vi "stop.vi"(3 "error in (no error)":errorcluster, 4 "stop":bool, 5 "HamegHMPSupply in":refnum<class "HamegHMPSupply.lvclass">) -> (0 "error out":errorcluster, 1 "Stopped":bool, 2 "HamegHMPSupply out":refnum<class "HamegHMPSupply.lvclass">)   [LabVIEW 2011, in "Hardware.lvlib" / "Channels.lvlib" / "HamegHMPSupply.lvclass"]
doc: "Abstract Method.\n\nStops the analog output. This vi indicates of the analog output has stopped, and can be used to actively stop the output."
uses:
  HamegHMPSupply.lvclass
  HamegHMPSupply.lvclass/HamegHMPSupply.ctl
  AnalogOutput.lvclass
  Tools/Filing/FileNeologist/FileNeologist.lvclass
  Tools/Filing.lvlib
panel:
  in  "measure":bool=TRUE
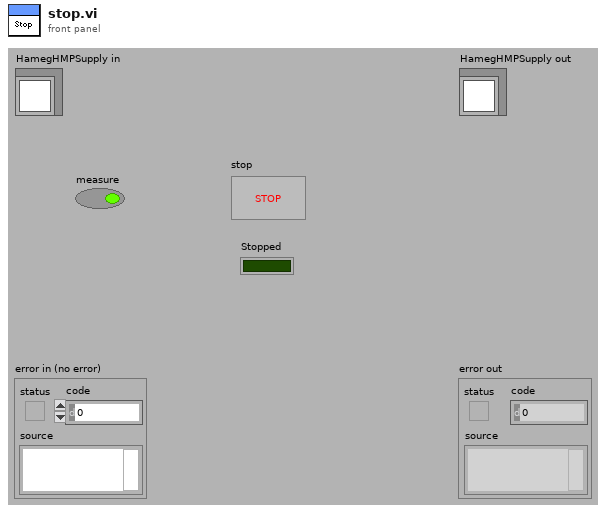
[diagram p1: front panel]
types:
  T1 = enum16{"open", "replace", "create", "open or create", "replace or create", "replace or create with confirmation"}
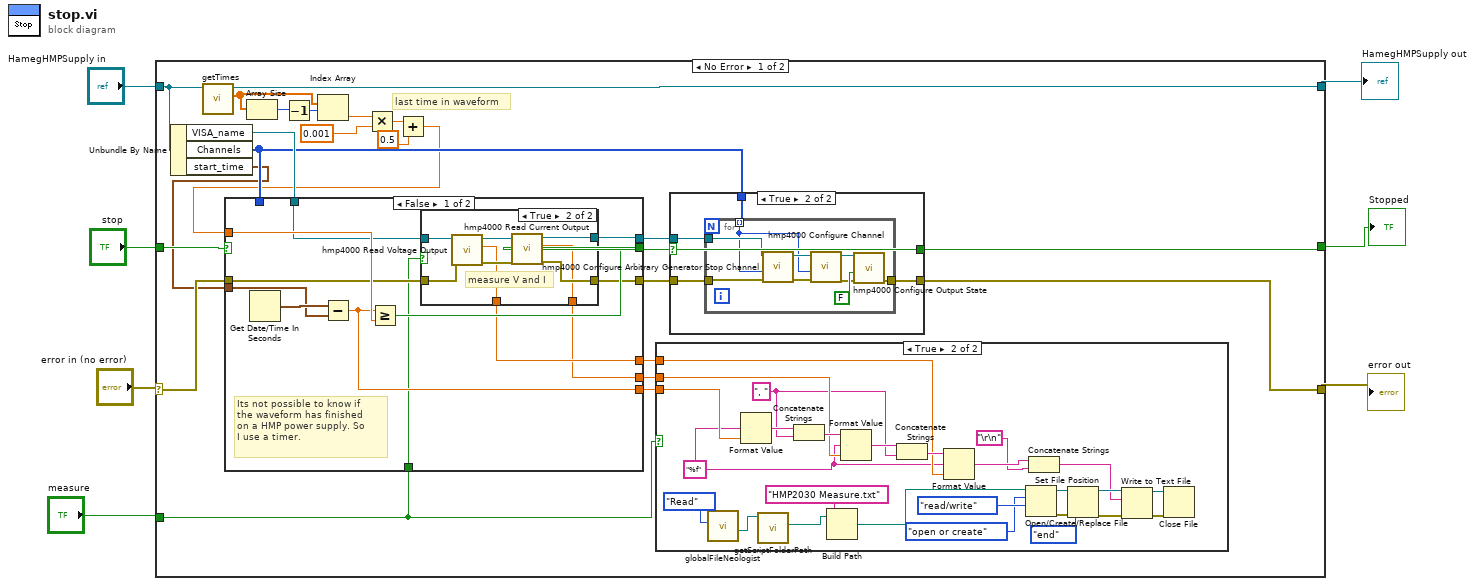
[diagram p0: block diagram]
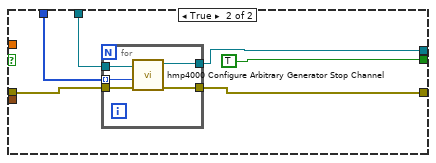
[diagram p5: hidden frame]
diagram:
  n1 = case shown="No Error" "error in (no error)" {
    selector: "error in (no error)" -> [w29 w107]
    tunnel: [w21 w109] -> w7
    tunnel: "HamegHMPSupply in" -> [w22 w109]
    tunnel: [w25 w107] -> w2
    tunnel: [w24 w108] -> w4
    tunnel: "stop" -> [w30 w108]
    tunnel: "measure" -> [w8 _]
    frame No Error {
      # "last time in waveform"
      n2 = Unbundle By Name(w22) -> ("VISA_name"=w31:refnum<visa-resource-name>, "Channels"=w23:i32[], "start_time"=w12:timestamp)
      n3 = call "getTimes.vi"("AnalogOutput in"=w22) -> ("times"=w18:dbl[], "AnalogOutput out"=w21:refnum<class "HamegHMPSupply.lvclass">)  [unwired: 8 in, 1 out]
      n4 = Array Size(array=w18) -> (size(s)=w20:i32)
      n5 = Decrement(x=w20) -> (x-1=w19:i32)
      n6 = Index Array(array=w18, index=w19) -> (element=w17:dbl)
      n7 = Multiply(x=w17, y=0.001) -> (x*y=w16:dbl)
      n8 = Add(x=w16, y=0.5) -> (x+y=w13:dbl)
      n9 = case shown="False" w30 {
        tunnel: w31 -> [w81 w101]
        tunnel: [w82 TRUE] -> w28
        tunnel: w23 -> [_ w100]
        tunnel: [w79 w99] -> w27
        tunnel: w29 -> [w78 w98]
        tunnel: [w80 w96] -> w26
        tunnel: w13 -> [w83 _]
        tunnel: w12 -> [w84 _]
        tunnel: [w77 _] -> w9
        tunnel: [w76 _] -> w10
        tunnel: [w75 _] -> w11
        tunnel: w8 -> [w74 _]
        frame False {
          # "Its not possible to know if\nthe waveform has finished\non a HMP power supply. So \nI use a timer."
          n10 = Get Date/Time In Seconds() -> (seconds since 1Jan1904=w85:timestamp)
          n11 = Subtract(x=w85, y=w84) -> (x-y=w75:dbl)
          n12 = Greater Or Equal?(x=w75, y=w83) -> (x >= y?=w82:bool)
          n13 = case shown="True" w74 {
            tunnel: w81 -> [w86 w93]
            tunnel: [w86 w92] -> w80
            tunnel: [w87 w91] -> w79
            tunnel: w78 -> [w87 w90]
            tunnel: [_ w89] -> w77
            tunnel: [_ w88] -> w76
            frame False {
            }
            frame True {
              # "measure V and I"
              n14 = call <instrlib>:"hmp4000 Read Voltage Output.vi"("error in (no error)"=w90, "VISA resource name"=w93) -> ("error out"=w94:errorcluster, "Voltage Value"=w89:dbl, "VISA resource name out"=w95:refnum<visa-resource-name>)  [unwired: 7 in]
              n15 = call <instrlib>:"hmp4000 Read Current Output.vi"("error in (no error)"=w94, "VISA resource name"=w95) -> ("error out"=w91:errorcluster, "Current Value"=w88:dbl, "VISA resource name out"=w92:refnum<visa-resource-name>)  [unwired: 7 in]
            }
          }
        }
        frame True {
          n16 = for {
            tunnel: w101 -> [w106]
            tunnel: w100 -> [w105] mode=indexing
            tunnel: [w104] -> w99
            tunnel: w98 -> [w103]
            tunnel: [w102] -> w96
            n17 = call <instrlib>:"hmp4000 Configure Arbitrary Generator Stop Channel.vi"("error in (no error)"=w103, "Channel (Channel 1)"=w105, "VISA resource name"=w106) -> ("error out"=w104:errorcluster, "VISA resource name out"=w102:refnum<visa-resource-name>)  [unwired: 7 in]
          }
        }
      }
      n18 = case shown="True" w8 {
        tunnel: w11 -> [_ w57]
        tunnel: w10 -> [_ w54]
        tunnel: w9 -> [_ w50]
        frame False {
        }
        frame True {
          w51 = ", "
          w49 = "%f"
          n19 = call "globalFileNeologist.vi"("Action"=enum16{"Write", "Read"}."Read") -> ("FileNeologist out"=w47:refnum<class "FileNeologist.lvclass">)  [unwired: 10 in]
          n20 = Format Value(format string=w49, value (0)=w57) -> (output string=w56:string)  [unwired: 1 in]
          n21 = call "getScriptFolderPath.vi"("FileNeologist in"=w47) -> ("Path"=w46:path)  [unwired: 8 in, 2 out]
          n22 = Concatenate Strings(w56, w51) -> (w55:string)
          n23 = Build Path(base path=w46, name or relative path="HMP2030 Measure.txt") -> (appended path=w44:path)
          n24 = Format Value(string ("")=w55, format string=w49, value (0)=w54) -> (output string=w52:string)
          n25 = Concatenate Strings(w52, w51) -> (w53:string)
          n26 = Format Value(string ("")=w53, format string=w49, value (0)=w50) -> (output string=w34:string)
          n27 = Open/Create/Replace File(file path (use dialog)=w44, operation (0:open)=T1."open or create", access (0:read/write)=enum16{"read/write", "read-only", "write-only"}."read/write") -> (refnum out=w41:refnum<file>, error out=w40:errorcluster)  [unwired: 3 in, 1 out]
          n28 = Concatenate Strings(w34, "\r\n") -> (w32:string)
          n29 = Set File Position(refnum=w41, from (0:start)=enum16{"start", "end", "current"}."end", error in=w40) -> (refnum out=w38:refnum<file>, error out=w37:errorcluster)  [unwired: 1 in]
          n30 = Write to Text File(file (use dialog)=w38, text=w32, error in=w37) -> (refnum out=w35:refnum<file>, error out=w36:errorcluster)  [unwired: 1 in, 1 out]
          n31 = Close File(refnum=w35, error in=w36) -> ()  [unwired: 2 out]
        }
      }
      n32 = case shown="True" w28 {
        selector: w28 -> [w59 w61]
        tunnel: w27 -> [w58 w64]
        tunnel: w26 -> [_ w63]
        tunnel: [w58 w62] -> w25
        tunnel: [w59 w61] -> w24
        tunnel: w23 -> [_ w60]
        frame False {
        }
        frame True {
          n33 = for {
            tunnel: w64 -> [w67]
            tunnel: w63 -> [w66]
            tunnel: [w72] -> w62
            tunnel: w60 -> [w65] mode=indexing
            n34 = call <instrlib>:"hmp4000 Configure Arbitrary Generator Stop Channel.vi"("error in (no error)"=w67, "Channel (Channel 1)"=w65, "VISA resource name"=w66) -> ("error out"=w68:errorcluster, "VISA resource name out"=w69:refnum<visa-resource-name>)  [unwired: 7 in]
            n35 = call <instrlib>:"hmp4000 Configure Channel.vi"("error in (no error)"=w68, "Channel (Channel 1)"=w65, "VISA resource name"=w69) -> ("error out"=w71:errorcluster, "VISA resource name out"=w70:refnum<visa-resource-name>)  [unwired: 7 in]
            n36 = call <instrlib>:"hmp4000 Configure Output State.vi"("error in (no error)"=w71, "Output State (Off)"=FALSE, "VISA resource name"=w70) -> ("error out"=w72:errorcluster)  [unwired: 7 in, 1 out]
          }
        }
      }
    }
    frame Error {
    }
  }
  "error out" <- w2
  "HamegHMPSupply out" <- w7
  "Stopped" <- w4
